vi "Initialize.vi"(7 "Plugin Name":string, 8 "error in":errorcluster, 9 "Compiled Settings":variant, 10 "iPluginAPI in":refnum<class "CustomDeviceAPI.lvclass">, 11 "CD In":refnum<class "Template.lvclass">) -> (0 "error out":errorcluster, 3 "CD out":refnum<class "Template.lvclass">)   [LabVIEW 2026, in "Template Plugin.lvlib" / "Template.lvclass"]
uses:
  Template.lvclass
  Template.lvclass/Template.ctl
  Processes/Template.Async.vi
  Types/TargetSettings.ctl
  Logging/Log.Debug.vi
  <userlib>/NIVS Inline Async API (Express)/_VS Inline Async API (Express)/VS Inline Async API (Express)/VS Inline Async API (Express).lvclass
  <userlib>/CustomDeviceInterfaces_v1.lvlibp/custom-device-express-framework/Source/Custom Device Interfaces/CustomDeviceAPI/CustomDeviceAPI.lvclass
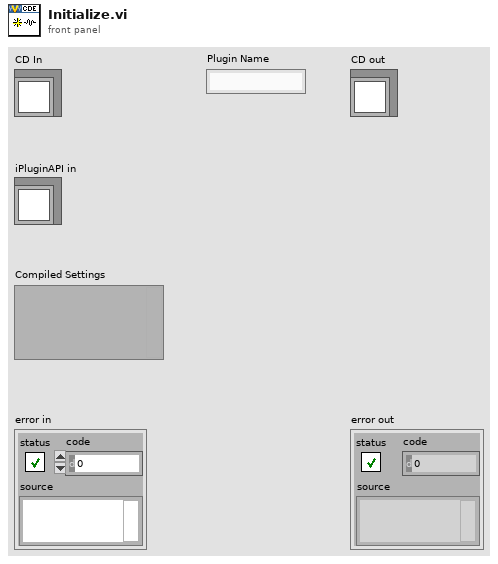
[diagram p1: front panel]
types:
  T1 = typedef "Template Plugin.lvlib/Template.lvclass/TargetSettings.ctl" = cluster{"Name":string}
  T2 = cluster{"Read":cluster{"Refs":cluster{"Data Reference":i32, "Offset":u64, "Length":u64}[], "Values":dbl[]}[], "Write":cluster{"Refs":cluster{"Data Reference":i32, "Offset":u64, "Length":u64}[], "Values":dbl[]}[], "ReadWrite":cluster{"Refs":i32[], "Values":dbl[], "Reset Values":dbl[]}[], "LUT":variant}
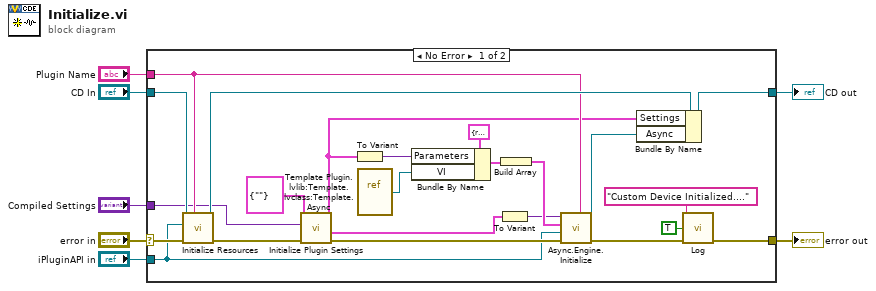
[diagram p0: block diagram]
diagram:
  n1 = case shown="No Error" "error in" {
    selector: "error in" -> [w30 w32]
    tunnel: "CD In" -> [w17 w31]
    tunnel: "iPluginAPI in" -> [w12 _]
    tunnel: [w25 w31] -> w3
    tunnel: [w28 w32] -> w6
    tunnel: "Compiled Settings" -> [w9 _]
    tunnel: "Plugin Name" -> [w18 _]
    frame No Error {
      n2 = call "Initialize Resources.vi"("Plugin Name"=w18, "error in"=w30, "CDAPI in"=w12, "CD in"=w17) -> ("error out"=w27:errorcluster, "CD out"=w23:refnum<class "Template.lvclass">)  [unwired: 6 in]
      n3 = call "Initialize Plugin Settings.vi"("error in"=w27, "Compiled Settings"=w9, "Plugin Engine Settings"=T1 {"Name"=""} ("Settings")) -> ("error out"=w26:errorcluster, "Channel Refs"=w8:T2, "Plugin Engine Settings"=w11:T1)  [unwired: 6 in]
      n4 = To Variant(anything=w11) -> (Variant=w14:variant)
      n5 = vi-ref "Template Plugin.lvlib:Template.lvclass:Template.Async.vi"() -> (w24:refnum<vi>)
      n6 = Bundle By Name(cluster=cluster{"VI":refnum<vi>, "Parameters":variant} {"VI"=refnum, "Parameters"=variant} ("Process"), "Parameters"=w14, "VI"=w24) -> (w21:cluster{"VI":refnum<vi>, "Parameters":variant})
      n7 = To Variant(anything=w8) -> (Variant=w13:variant)
      n8 = Build Array(w21) -> (w20:cluster{"VI":refnum<vi>, "Parameters":variant}[])
      n9 = call <userlib>:"Async.Engine.Initialize.vi"("Custom Device Name"=w18, "error in"=w26, "CDAPI"=w12, "Processes"=w20, "Compiled.InlineAsync.Settings"=w13) -> ("error out"=w29:errorcluster, "Async out"=w19:refnum<class "VS Inline Async API (Express).lvclass">)  [unwired: 5 in]
      n10 = Bundle By Name(cluster=w23, "Settings"=w11, "Async"=w19) -> (w25:refnum<class "Template.lvclass">)
      n11 = call-poly "Log.vi"("error in"=w29, "Add to log file? (F)"=TRUE, "Message"="Custom Device Initialized....") -> ("error out"=w28:errorcluster)  [unwired: 8 in]
    }
    frame Error {
    }
  }
  "error out" <- w6
  "CD out" <- w3
